vi "Wash Needle Impl.vi"(8 "error in (no error)":errorcluster, 11 "Simulated Autosampler in":refnum<class "Simulated Autosampler.lvclass">) -> (0 "error out":errorcluster, 3 "Simulated Autosampler out":refnum<class "Simulated Autosampler.lvclass">)   [LabVIEW 2023, in "Simulated Autosampler.lvlib" / "Simulated Autosampler.lvclass"]
uses:
  Simulated Autosampler.lvclass
  Simulated Autosampler.lvclass/Simulated Autosampler.ctl
  Autosampler/Autosampler.lvclass
  Autosampler/Autosampler State.ctl
  Autosampler/Autosampler.lvlib
  C:/FLASH/Development/Hardware/Autosampler/Autosampler.lvclass
  C:/FLASH/Development/Hardware/Device/Device.lvclass
  C:/Program Files/National Instruments/LabVIEW 2023/vi.lib/ActorFramework/Actor/Actor.lvclass
  C:/FLASH/Development/Hardware/Simulated Autosampler/Simulated Autosampler.lvclass
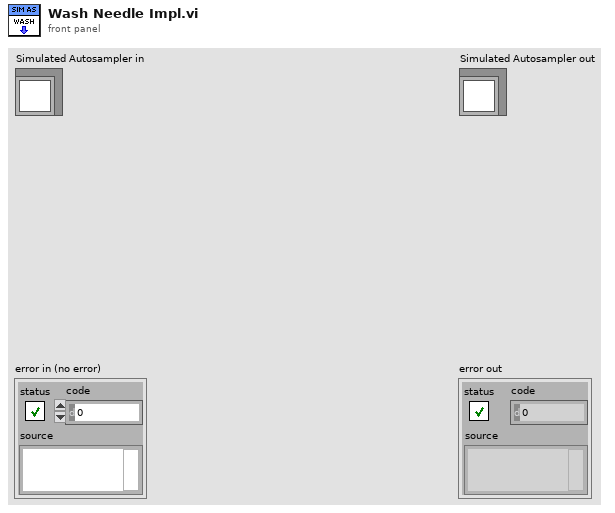
[diagram p1: front panel]
types:
  T1 = typedef "Autosampler.lvlib/Autosampler State.ctl" = enum16{"Ready", "Injection", "Washing", "Shaking", "Getting Ready", "Error"}
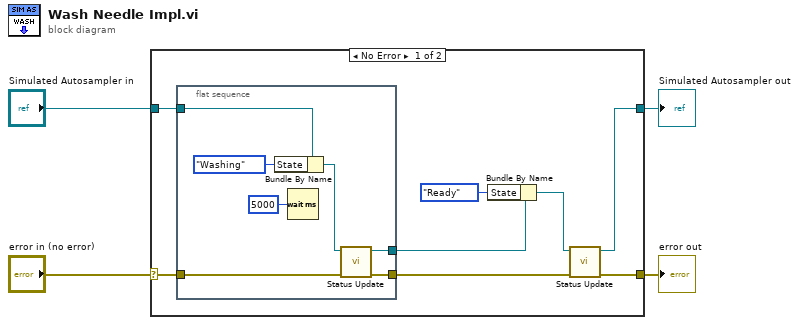
[diagram p0: block diagram]
diagram:
  n1 = case shown="No Error" "error in (no error)" {
    selector: "error in (no error)" -> [w11 w20]
    tunnel: [w10 w20] -> w3
    tunnel: "Simulated Autosampler in" -> [w12 w21]
    tunnel: [w9 w21] -> w1
    frame No Error {
      n2 = flat-sequence {
        tunnel: w12 -> [w17]
        tunnel: w11 -> [w19]
        tunnel: [w16] -> w6
        tunnel: [w18] -> w5
        frame #0 {
          n3 = Bundle By Name(cluster=w17, "State"=Autosampler_State."Washing" ("Autosampler Status.State")) -> (w15:refnum<class "Simulated Autosampler.lvclass">)
          n4 = Wait (ms)(milliseconds to wait=u32 5000) -> ()  [unwired: 1 out]
          n5 = call "Status Update.vi"("error in (no error)"=w19, "Autosampler in"=w15) -> ("error out"=w18:errorcluster, "Autosampler out"=w16:refnum<class "Simulated Autosampler.lvclass">)  [unwired: 7 in, 1 out]
        }
      }
      n6 = Bundle By Name(cluster=w6, "State"=Autosampler_State."Ready" ("Autosampler Status.State")) -> (w7:refnum<class "Simulated Autosampler.lvclass">)
      n7 = call "Status Update.vi"("error in (no error)"=w5, "Autosampler in"=w7) -> ("error out"=w10:errorcluster, "Autosampler out"=w9:refnum<class "Simulated Autosampler.lvclass">)  [unwired: 7 in, 1 out]
    }
    frame Error {
    }
  }
  "error out" <- w3
  "Simulated Autosampler out" <- w1
